vi "Create Events.vi"() -> (2 "Event Registration Refnum":refnum<event-registration>, 3 "output cluster":T1)   [LabVIEW 2021]
uses:
  <vilib>/MakerHub/PS4-Controller/Private/Type Defs/Indicators/Slider.ctl
  <vilib>/MakerHub/PS4-Controller/LMH-PS4.lvlib
  <vilib>/MakerHub/PS4-Controller/Private/Type Defs/Indicators/Dpad.ctl
  <vilib>/MakerHub/PS4-Controller/Private/Type Defs/Indicators/Pad_Button.ctl
  <vilib>/MakerHub/PS4-Controller/Private/Type Defs/Indicators/PS.ctl
  <vilib>/MakerHub/PS4-Controller/Private/Type Defs/Indicators/Options.ctl
  <vilib>/MakerHub/PS4-Controller/Private/Type Defs/Indicators/Share.ctl
  <vilib>/MakerHub/PS4-Controller/Private/Type Defs/Indicators/R1.ctl
  <vilib>/MakerHub/PS4-Controller/Private/Type Defs/Indicators/L1.ctl
  <vilib>/MakerHub/PS4-Controller/Private/Type Defs/Indicators/Triangle.ctl
  <vilib>/MakerHub/PS4-Controller/Private/Type Defs/Indicators/Circle.ctl
  <vilib>/MakerHub/PS4-Controller/Private/Type Defs/Indicators/X.ctl
  <vilib>/MakerHub/PS4-Controller/Private/Type Defs/Indicators/Square.ctl
  <vilib>/MakerHub/PS4-Controller/Private/Type Defs/Indicators/Controller.ctl
  event cluster.ctl
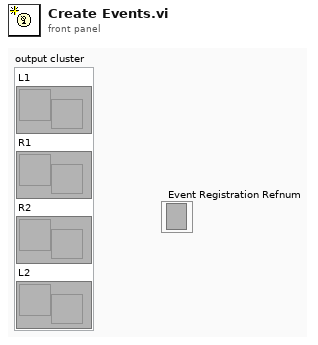
[diagram p1: front panel]
types:
  T1 = typedef "event cluster.ctl" = cluster{"L1":refnum<user-event>, "R1":refnum<user-event>, "R2":refnum<user-event>, "L2":refnum<user-event>}
  T2 = typedef "LMH-PS4.lvlib/Controller.ctl" = cluster{"Square Button":T3, "X Button":T4, "Circle Button":T5, "Triangle Button":T6, "L1":T7, "R1":T8, "Share Button":T9, "Options Button":T10, "PS Button":T11, "Pad Button":T12, "D-Pad":T13, "L2":T14, "R2":T14, "Thumbstick_Left":cluster{i32[], i32[]}, "Thumbstick_Right":cluster{i32[], i32[]}}
  T3 = typedef "LMH-PS4.lvlib/Square.ctl" = bool
  T4 = typedef "LMH-PS4.lvlib/X.ctl" = bool
  T5 = typedef "LMH-PS4.lvlib/Circle.ctl" = bool
  T6 = typedef "LMH-PS4.lvlib/Triangle.ctl" = bool
  T7 = typedef "LMH-PS4.lvlib/L1.ctl" = bool
  T8 = typedef "LMH-PS4.lvlib/R1.ctl" = bool
  T9 = typedef "LMH-PS4.lvlib/Share.ctl" = bool
  T10 = typedef "LMH-PS4.lvlib/Options.ctl" = bool
  T11 = typedef "LMH-PS4.lvlib/PS.ctl" = bool
  T12 = typedef "LMH-PS4.lvlib/Pad_Button.ctl" = bool
  T13 = typedef "LMH-PS4.lvlib/Dpad.ctl" = u16
  T14 = typedef "LMH-PS4.lvlib/Slider.ctl" = i32
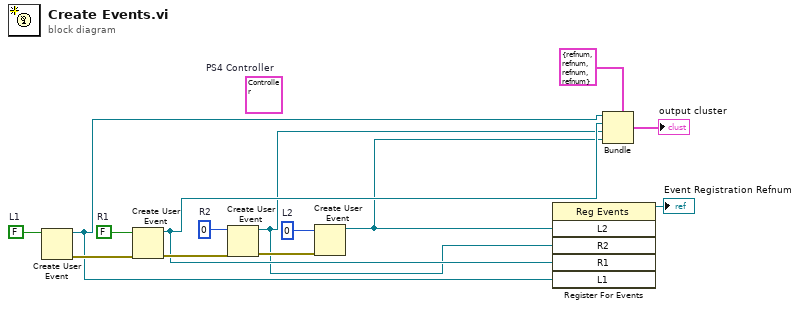
[diagram p0: block diagram]
diagram:
  w9 = FALSE  # L1
  w8 = FALSE  # R1
  w11 = 0  # R2
  w10 = 0  # L2
  (unwired) T2 {"Square Button"=FALSE, "X Button"=FALSE, "Circle Button"=FALSE, "Triangle Button"=FALSE, "L1"=FALSE, "R1"=FALSE, "Share Button"=FALSE, "Options Button"=FALSE, "PS Button"=FALSE, "Pad Button"=FALSE, "D-Pad"=5, "L2"=0, "R2"=0, "Thumbstick_Left"={[], []}, "Thumbstick_Right"={[], []}}  # PS4 Controller
  n1 = Create User Event(user event datatype=w9) -> (user event=w7:refnum<user-event>, error out=w13:errorcluster)  [unwired: 1 in]
  n2 = Create User Event(user event datatype=w8, error in=w13) -> (user event=w6:refnum<user-event>, error out=w14:errorcluster)
  n3 = Create User Event(user event datatype=w11, error in=w14) -> (user event=w5:refnum<user-event>, error out=w12:errorcluster)
  n4 = Create User Event(user event datatype=w10, error in=w12) -> (user event=w4:refnum<user-event>)  [unwired: 1 out]
  n5 = register-events(w4, w5, w6, w7) -> (reference out=→"Event Registration Refnum":refnum<event-registration>)  [unwired: 2 in, 1 out]
  n6 = Bundle(cluster=T1 {"L1"=refnum, "R1"=refnum, "R2"=refnum, "L2"=refnum} ("output cluster 2"), "L1"=w7, "R1"=w6, "R2"=w5, "L2"=w4) -> (→"output cluster":T1)
